vi "Insight_CMD_composer.vi"(6 "Mode (Read / Write)":enum8{"Write", "Read"}(ring)=enum."Read", 7 "Parameter Type":enum16{"Value", "MAXimum", "MINimum", "DEFault"}(ring), 8 "error in (no error)":errorcluster, 9 "Value":dbl, 10 "CMD":string, 11 "String Format":string=" %f") -> (0 "error out":errorcluster, 2 "Command String":string)   [LabVIEW 2015]
doc: "Insight Photonic Solutions\n\nThis VI composes the string to send to the laser when writing or reading the value of a numeric parameter. Command strings may be selected as either Read or Write. Commands to the laser may explicitly set a numeric value for a parameter, or may use the keywords MAXimum, MINimum or DEFault to set the parameter to any of these 3 special case values. The command string is composed for all 8 of these cases.\n\nUse this VI to prepare the string sent into the Insight Telnet Communication VI.\n\nINPUTS\n\nCMD - The SCPI command for reading or writing the parameter of interest. (Default = empty string).\nMode - Tells the VI whether the command is a Read or a Write. (Default = Read).\nParameter Type - Tells the VI whether the command should use a Value or a keyword MAXimum, MINimum or DEFault to set the parameter value. (Default = Value).\nValue - The numeric value to set the parameter. (Default = 0).\nString Format - The format string for the Scan into String that formats the Value appended to the CMD string. (Default = \\s%f).\nerror in - The standard LabView Error cluster. Use this to enforce sequentiality and error tracking.\n\nOUTPUT\n\nCommand String - The completed command string including the CMD string, the Value or keyword, and ? if a Read.\nerror out - The standard LabView Error cluster. Reports error in composing the Command String, or passes through any errors prior to this VI.\n\nver 1.0 - original release"
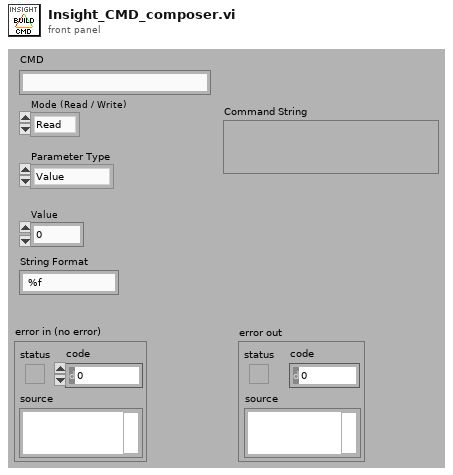
[diagram p1: front panel]
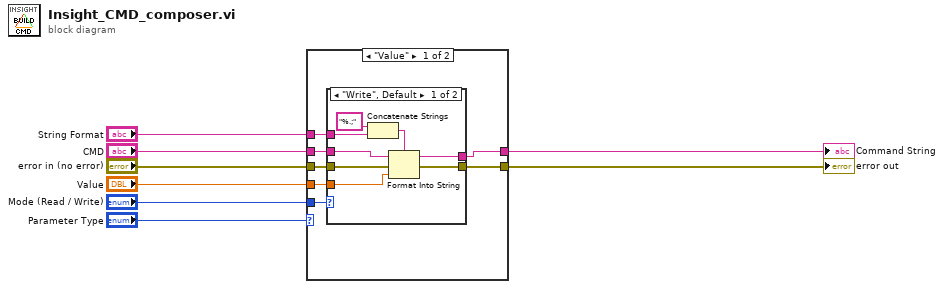
[diagram p0: block diagram]
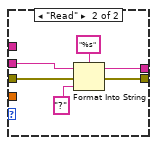
[diagram p2: hidden frame]
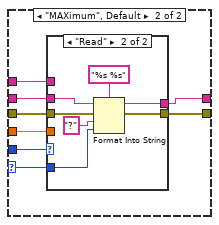
[diagram p3: hidden frame]
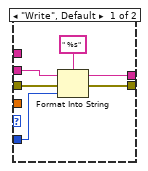
[diagram p4: hidden frame]
diagram:
  n1 = case shown="\"Value\"" "Parameter Type" {
    selector: "Parameter Type" -> [_ w30]
    tunnel: "Mode (Read / Write)" -> [w15 w37]
    tunnel: "error in (no error)" -> [w14 w36]
    tunnel: [w13 w35] -> w6
    tunnel: "CMD" -> [w12 w34]
    tunnel: [w11 w33] -> w4
    tunnel: "String Format" -> [w10 w32]
    tunnel: "Value" -> [w9 w31]
    frame "Value" {
      n2 = case shown="\"Write\", Default" w15 {
        tunnel: [w23 w25] -> w13
        tunnel: w14 -> [w22 w24]
        tunnel: w12 -> [w21 w27]
        tunnel: [w20 w26] -> w11
        tunnel: w10 -> [w18 _]
        tunnel: w9 -> [w19 _]
        frame "Write", Default {
          n3 = Concatenate Strings("%.;" ("string"), w18) -> (w17:string)
          n4 = Format Into String(format string=w17, initial string=w21, error in=w22, w19) -> (resulting string=w20:string, error out=w23:errorcluster)
        }
        frame "Read" {
          n5 = Format Into String(format string="%s", initial string=w27, error in=w24, "?" ("input 1")) -> (resulting string=w26:string, error out=w25:errorcluster)
        }
      }
    }
    frame "MAXimum", Default {
      n6 = case shown="\"Read\"" w37 {
        tunnel: [w43 w46] -> w35
        tunnel: w36 -> [w42 w45]
        tunnel: w34 -> [w41 w48]
        tunnel: [w40 w47] -> w33
        tunnel: w32 -> [_ _]
        tunnel: w31 -> [_ _]
        tunnel: w30 -> [w38 w44]
        frame "Write", Default {
          n7 = Format Into String(format string=" %s", initial string=w41, error in=w42, w38) -> (resulting string=w40:string, error out=w43:errorcluster)
        }
        frame "Read" {
          n8 = Format Into String(format string="%s %s", initial string=w48, error in=w45, "?" ("input 1"), w44) -> (resulting string=w47:string, error out=w46:errorcluster)
        }
      }
    }
  }
  "error out" <- w6
  "Command String" <- w4
